vi "test Source.vi"(8 "error in (no error)":errorcluster, 11 "TestCase in":refnum<class "Parameter Setting.lvclass">) -> (0 "error out":errorcluster, 3 "TestCase out":refnum<class "Parameter Setting.lvclass">)   [LabVIEW 2020, in "Static Errors Tests.lvlib" / "Parameter Setting.lvclass"]
uses:
  Parameter Setting.lvclass
  Parameter Setting.lvclass/Parameter Setting.ctl
  C:/Program Files/National Instruments/LabVIEW 2027/vi.lib/addons/_JKI Toolkits/VI Tester/TestCase.llb/TestCase.lvclass
  <vilib>/addons/_JKI Toolkits/VI Tester/TestCase.llb/TestCase.lvclass
  Static Errors.lvlib
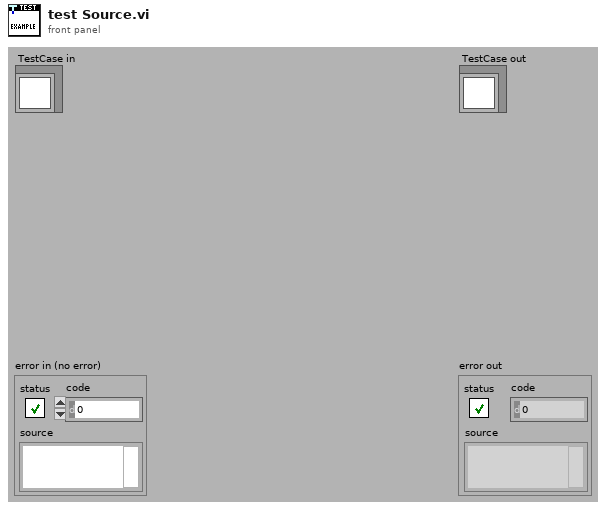
[diagram p1: front panel]
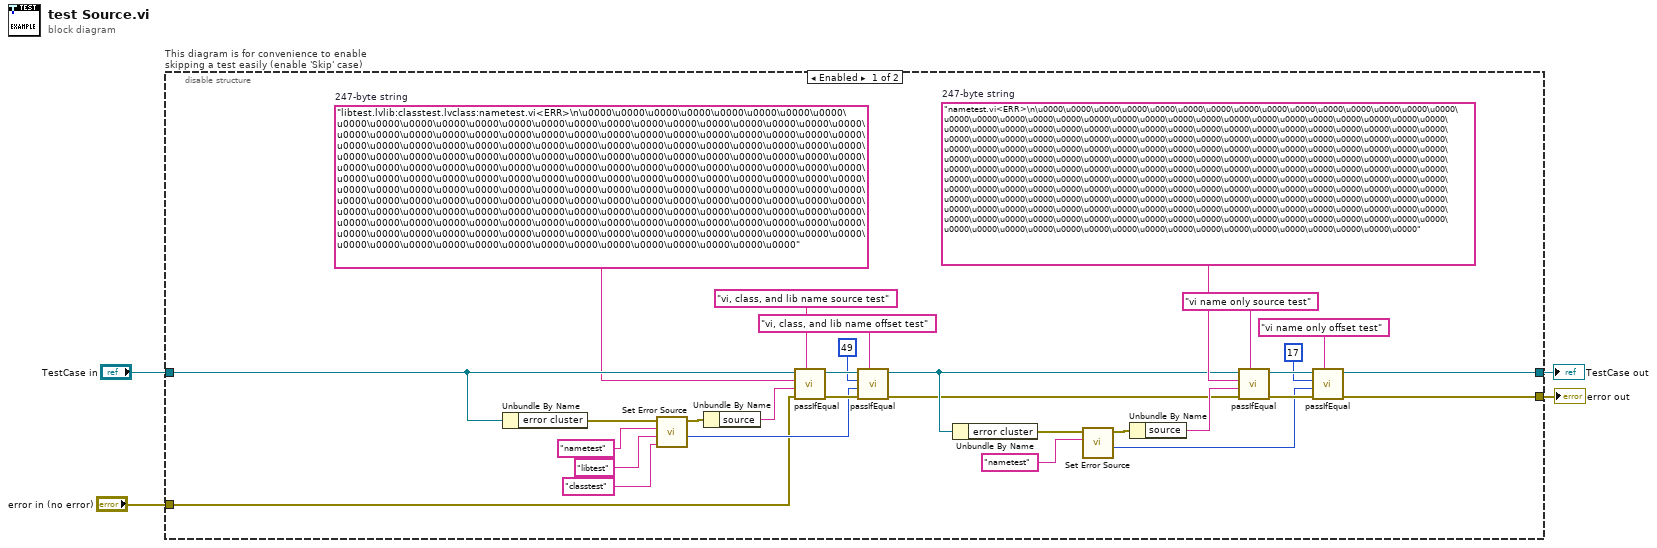
[diagram p0: block diagram]
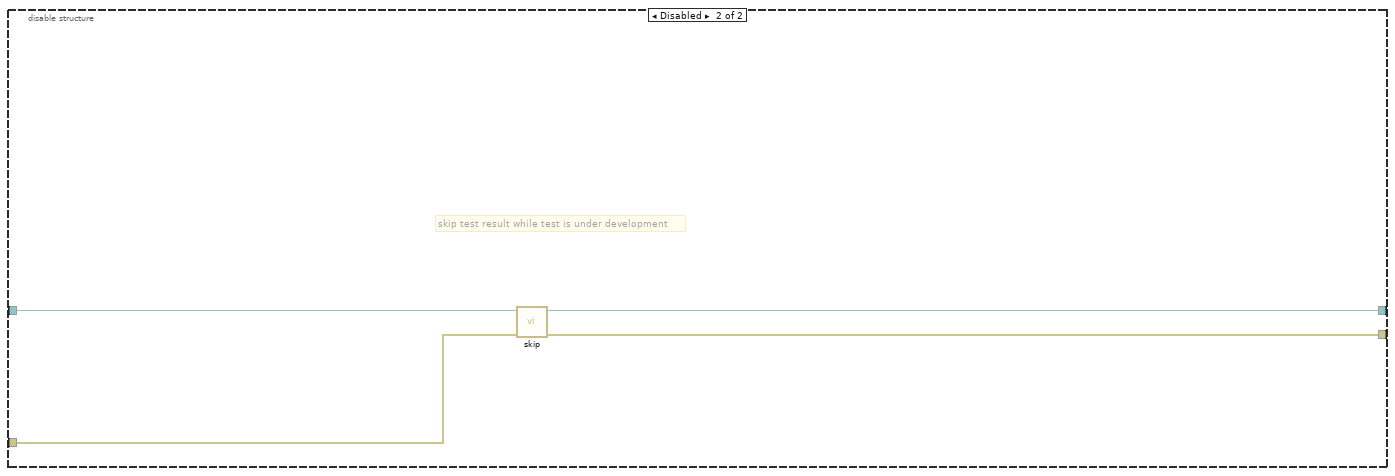
[diagram p2: hidden frame]
diagram:
  n1 = disable-structure "This diagram is for convenience to enable skipping a test easily (enable 'Skip' case)" shown="Enabled" {
    disable-tunnel: "TestCase in" -> [w34 w38]
    disable-tunnel: [w16 w36] -> w2
    disable-tunnel: [w15 w37] -> w1
    disable-tunnel: "error in (no error)" -> [w6 w35]
    frame Enabled {
      w23 = "nametest.vi<ERR>\n\u0000\u0000\u0000\u0000\u0000\u0000\u0000\u0000\u0000\u0000\u0000\u0000\u0000\u0000\u0000\u0000\u0000\u0000\u0000\u0000\u0000\u0000\u0000\u0000\u0000\u0000\u0000\u0000\u0000\u0000\u0000\u0000\u0000\u0000\u0000\u0000\u0000\u0000\u0000\u0000\u0000\u0000\u0000\u0000\u0000\u0000\u0000\u0000\u0000\u0000\u0000\u0000\u0000\u0000\u0000\u0000\u0000\u0000\u0000\u0000\u0000\u0000\u0000\u0000\u0000\u0000\u0000\u0000\u0000\u0000\u0000\u0000\u0000\u0000\u0000\u0000\u0000\u0000\u0000\u0000\u0000\u0000\u0000\u0000\u0000\u0000\u0000\u0000\u0000\u0000\u0000\u0000\u0000\u0000\u0000\u0000\u0000\u0000\u0000\u0000\u0000\u0000\u0000\u0000\u0000\u0000\u0000\u0000\u0000\u0000\u0000\u0000\u0000\u0000\u0000\u0000\u0000\u0000\u0000\u0000\u0000\u0000\u0000\u0000\u0000\u0000\u0000\u0000\u0000\u0000\u0000\u0000\u0000\u0000\u0000\u0000\u0000\u0000\u0000\u0000\u0000\u0000\u0000\u0000\u0000\u0000\u0000\u0000\u0000\u0000\u0000\u0000\u0000\u0000\u0000\u0000\u0000\u0000\u0000\u0000\u0000\u0000\u0000\u0000\u0000\u0000\u0000\u0000\u0000\u0000\u0000\u0000\u0000\u0000\u0000\u0000\u0000\u0000\u0000\u0000\u0000\u0000\u0000\u0000\u0000\u0000\u0000\u0000\u0000\u0000\u0000\u0000\u0000\u0000\u0000\u0000\u0000\u0000\u0000\u0000\u0000\u0000\u0000\u0000\u0000\u0000\u0000\u0000\u0000\u0000\u0000\u0000\u0000\u0000\u0000\u0000\u0000\u0000\u0000\u0000\u0000\u0000\u0000\u0000\u0000\u0000\u0000\u0000\u0000\u0000"  # 247-byte string
      w24 = "libtest.lvlib:classtest.lvclass:nametest.vi<ERR>\n\u0000\u0000\u0000\u0000\u0000\u0000\u0000\u0000\u0000\u0000\u0000\u0000\u0000\u0000\u0000\u0000\u0000\u0000\u0000\u0000\u0000\u0000\u0000\u0000\u0000\u0000\u0000\u0000\u0000\u0000\u0000\u0000\u0000\u0000\u0000\u0000\u0000\u0000\u0000\u0000\u0000\u0000\u0000\u0000\u0000\u0000\u0000\u0000\u0000\u0000\u0000\u0000\u0000\u0000\u0000\u0000\u0000\u0000\u0000\u0000\u0000\u0000\u0000\u0000\u0000\u0000\u0000\u0000\u0000\u0000\u0000\u0000\u0000\u0000\u0000\u0000\u0000\u0000\u0000\u0000\u0000\u0000\u0000\u0000\u0000\u0000\u0000\u0000\u0000\u0000\u0000\u0000\u0000\u0000\u0000\u0000\u0000\u0000\u0000\u0000\u0000\u0000\u0000\u0000\u0000\u0000\u0000\u0000\u0000\u0000\u0000\u0000\u0000\u0000\u0000\u0000\u0000\u0000\u0000\u0000\u0000\u0000\u0000\u0000\u0000\u0000\u0000\u0000\u0000\u0000\u0000\u0000\u0000\u0000\u0000\u0000\u0000\u0000\u0000\u0000\u0000\u0000\u0000\u0000\u0000\u0000\u0000\u0000\u0000\u0000\u0000\u0000\u0000\u0000\u0000\u0000\u0000\u0000\u0000\u0000\u0000\u0000\u0000\u0000\u0000\u0000\u0000\u0000\u0000\u0000\u0000\u0000\u0000\u0000\u0000\u0000\u0000\u0000\u0000\u0000\u0000\u0000\u0000\u0000\u0000\u0000\u0000\u0000\u0000\u0000\u0000\u0000\u0000\u0000\u0000\u0000\u0000\u0000"  # 247-byte string
      n2 = Unbundle By Name(w34) -> ("error cluster"=w33:errorcluster)
      n3 = call "Set Error Source.vi"("class name (\"\")"="classtest", "library name (\"\")"="libtest", "vi name"="nametest", "error in"=w33) -> ("initial offset"=w14:i32, "error out"=w32:errorcluster)  [unwired: 6 in]
      n4 = Unbundle By Name(w32) -> ("source"=w25:string)
      n5 = call-dynamic "passIfEqual.vi"("custom report message (\"\")"="vi, class, and lib name source test" ("custom report message (\"\")"), "error in (no error)"=w6, "y"=w25, "x"=w24, "TestCase in"=w34) -> ("error out"=w21:errorcluster, "TestCase out"=w22:refnum<class "Parameter Setting.lvclass">)  [unwired: 5 in]
      n6 = call-dynamic "passIfEqual.vi"("custom report message (\"\")"="vi, class, and lib name offset test" ("custom report message (\"\")"), "error in (no error)"=w21, "y"=w14, "x"=49 ("new offset"), "TestCase in"=w22) -> ("error out"=w19:errorcluster, "TestCase out"=w20:refnum<class "Parameter Setting.lvclass">)  [unwired: 5 in]
      n7 = Unbundle By Name(w20) -> ("error cluster"=w28:errorcluster)
      n8 = call "Set Error Source.vi"("vi name"="nametest", "error in"=w28) -> ("initial offset"=w11:i32, "error out"=w29:errorcluster)  [unwired: 8 in]
      n9 = Unbundle By Name(w29) -> ("source"=w27:string)
      n10 = call-dynamic "passIfEqual.vi"("custom report message (\"\")"="vi name only source test" ("custom report message (\"\")"), "error in (no error)"=w19, "y"=w27, "x"=w23, "TestCase in"=w20) -> ("error out"=w17:errorcluster, "TestCase out"=w18:refnum<class "Parameter Setting.lvclass">)  [unwired: 5 in]
      n11 = call-dynamic "passIfEqual.vi"("custom report message (\"\")"="vi name only offset test" ("custom report message (\"\")"), "error in (no error)"=w17, "y"=w11, "x"=17 ("new offset"), "TestCase in"=w18) -> ("error out"=w15:errorcluster, "TestCase out"=w16:refnum<class "Parameter Setting.lvclass">)  [unwired: 5 in]
    }
    frame Disabled {
      # "skip test result while test is under development"
      n12 = call <vilib>:"skip.vi"("error in (no error)"=w35, "TestCase in"=w38) -> ("error out"=w37:errorcluster, "TestCase out"=w36:refnum<class "Parameter Setting.lvclass">)  [unwired: 8 in]
    }
  }
  "error out" <- w1
  "TestCase out" <- w2
